vi "Run Installer.vi"(8 "error in":errorcluster, 11 "installer path in":path) -> (0 "error out":errorcluster, 3 "installer path out":path)   [LabVIEW 2018]
uses:
  <vilib>/Utility/config.llb/Write Key (I32).vi
  <vilib>/Utility/config.llb/NI_LVConfig.lvlib
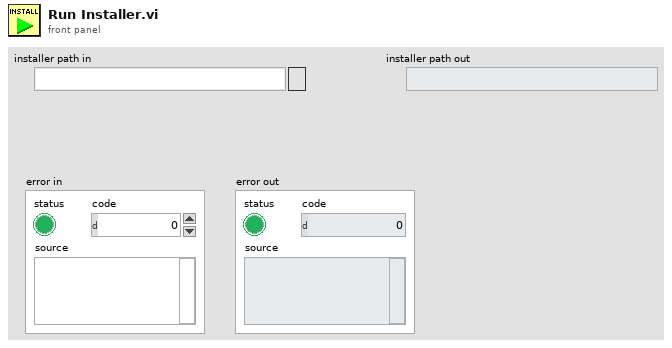
[diagram p1: front panel]
types:
  T1 = typedef "NI_LVConfig.lvlib/Config Data RefNum.ctl" = refnum<k1>
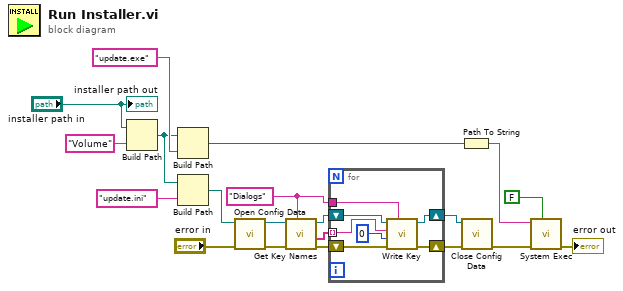
[diagram p0: block diagram]
diagram:
  w3 = "Dialogs" ("section")
  n1 = Build Path(base path="installer path in", name or relative path="Volume") -> (appended path=w14:path)
  n2 = Build Path(base path=w14, name or relative path="update.exe") -> (appended path=w17:path)
  n3 = Build Path(base path=w14, name or relative path="update.ini") -> (appended path=w13:path)
  n4 = call <vilib>:"Open Config Data.vi"("error in (no error)"="error in", "configuration file path"=w13) -> ("error out"=w7:errorcluster, "refnum"=w10:T1)  [unwired: 7 in, 1 out]
  n5 = call <vilib>:"Get Key Names.vi"("section"=w3, "error in (no error)"=w7, "refnum"=w10) -> ("error out"=w8:errorcluster, "key names"=w6:string[], "refnum out"=w9:T1)  [unwired: 5 in, 1 out]
  n6 = for {
    shift-right: [w26] -> w12
    shift-left: w9 -> [w27]
    shift-right: [w25] -> w11
    shift-left: w8 -> [w24]
    tunnel: w6 -> [w23] mode=indexing
    tunnel: w3 -> [w22]
    n7 = call-poly <vilib>:"Write Key.vi"("section"=w22, "error in (no error)"=w24, "value"=0, "key"=w23, "refnum"=w27) -> ("error out"=w25:errorcluster, "refnum out"=w26:T1)  [unwired: 4 in, 1 out]
  }
  n8 = Path To String(path=w17) -> (string=w16:string)
  n9 = call <vilib>:"Close Config Data.vi"("error in (no error)"=w11, "refnum"=w12) -> ("error out"=w4:errorcluster)  [unwired: 8 in, 1 out]
  n10 = call <vilib>:"System Exec.vi"("wait until completion? (T)"=FALSE, "error in (no error)"=w4, "command line"=w16) -> ("error out"=→"error out":errorcluster)  [unwired: 5 in, 3 out]
  "installer path out" <- "installer path in"
